vi "RP Read Temperature.vi"   [LabVIEW 2019]
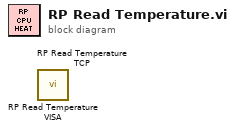
[diagram p0: block diagram]
diagram:
  n1 = call "RP Read Temperature VISA.vi"() -> ()  [unwired: 9 in, 3 out]
  n2 = call "RP Read Temperature TCP.vi"() -> ()  [unwired: 9 in, 3 out]
